vi "Read declination.vi"(8 "error in (no error)":errorcluster, 11 "RADecParameters in":refnum<class "RADecParameters.lvclass">) -> (0 "error out":errorcluster, 2 "Declination.lvclass":refnum<class "Declination.lvclass">, 3 "RADecParameters out":refnum<class "RADecParameters.lvclass">)   [LabVIEW 2014, in "TCSDataDefinitions.lvlib" / "TCSCommand.lvlib" / "TargetConfiguration.lvlib" / "Target.lvlib" / "FixedTarget.lvlib" / "RADecParameters.lvclass"]
uses:
  RADecParameters.lvclass
  Declination/Declination.lvclass
  RADecParameters.lvclass/RADecParameters.ctl
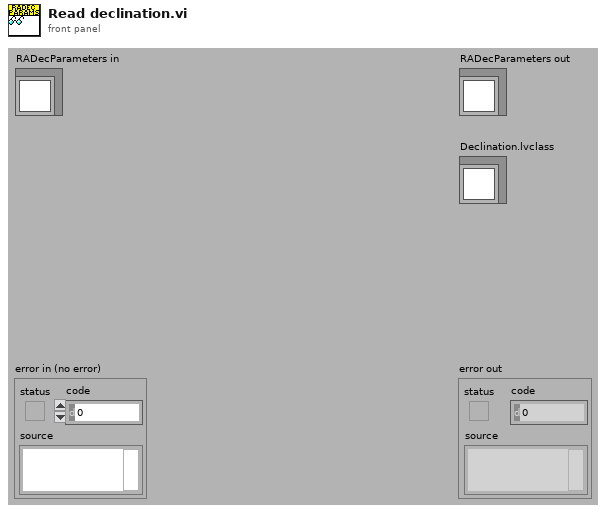
[diagram p1: front panel]
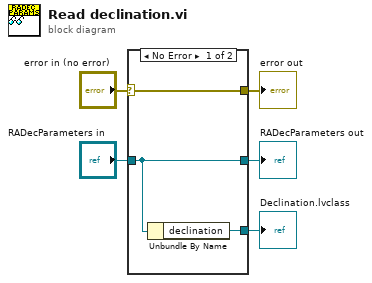
[diagram p0: block diagram]
diagram:
  n1 = case shown="No Error" "error in (no error)" {
    selector: "error in (no error)" -> [w8 w9]
    tunnel: [w8 w9] -> w4
    tunnel: [w7 w10] -> w2
    tunnel: "RADecParameters in" -> [w7 w10]
    tunnel: [w6 _] -> w1
    frame No Error {
      n2 = Unbundle By Name(w7) -> ("declination"=w6:refnum<class "Declination.lvclass">)
    }
    frame Error {
    }
  }
  "error out" <- w4
  "RADecParameters out" <- w2
  "Declination.lvclass" <- w1
